vi "Coward.vi"(8 "error in (no error)":errorcluster, 10 "Map":i32[](array[numeric]), 11 "Mother In":refnum<class "Mother.lvclass">) -> (0 "error out":errorcluster, 1 "Direction":T1, 2 "Action":T2, 3 "Mother Out":refnum<class "Mother.lvclass">, 4 "Replicated":refnum<class "Runner.lvclass">)   [LabVIEW 2014, in "Mother.lvclass"]
uses:
  Mother.lvclass
  Action Enum.ctl
  Direction Enum.ctl
  Runner.lvclass
  Coward/Coward.lvclass
  Attack Options.ctl
  Mother.lvclass/Mother.ctl
  SquareBattle.lvclass
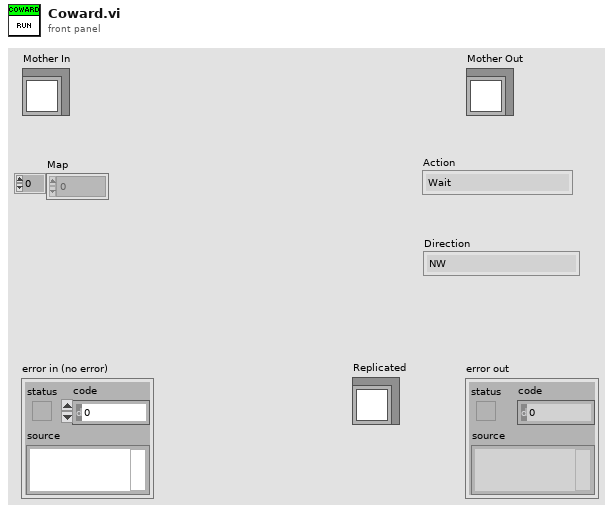
[diagram p1: front panel]
types:
  T1 = typedef "SquareBattle.lvclass/Direction Enum.ctl" = enum16{"NW", "N", "NE", "E", "SE", "S", "SW", "W"}
  T2 = typedef "SquareBattle.lvclass/Action Enum.ctl" = enum16{"Wait", "Move", "Attack", "Replicate"}
  T3 = typedef "Mother.lvclass/Attack Options.ctl" = enum16{"Attack", "Run", "Distract"}
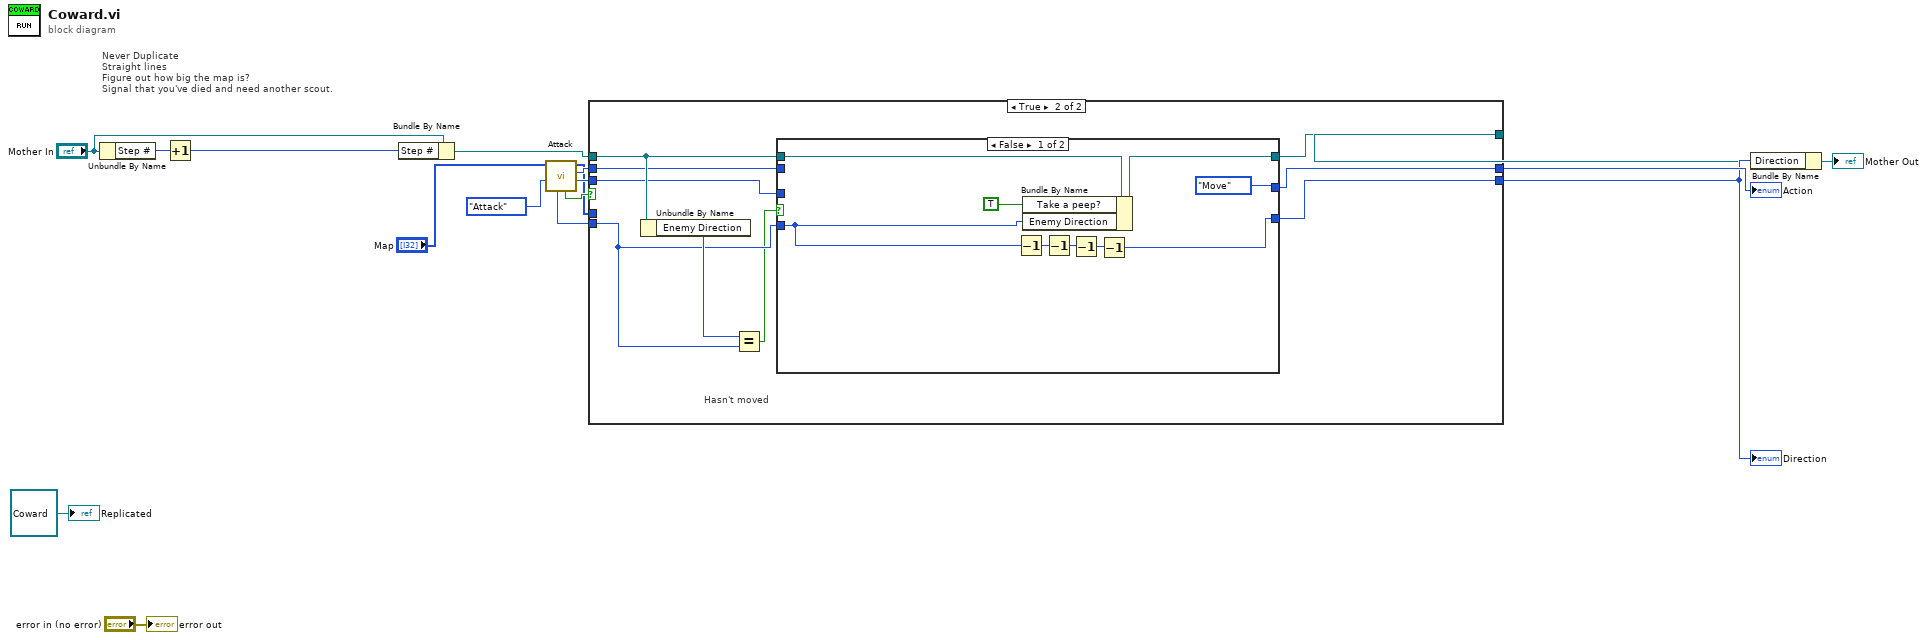
[diagram p0: block diagram]
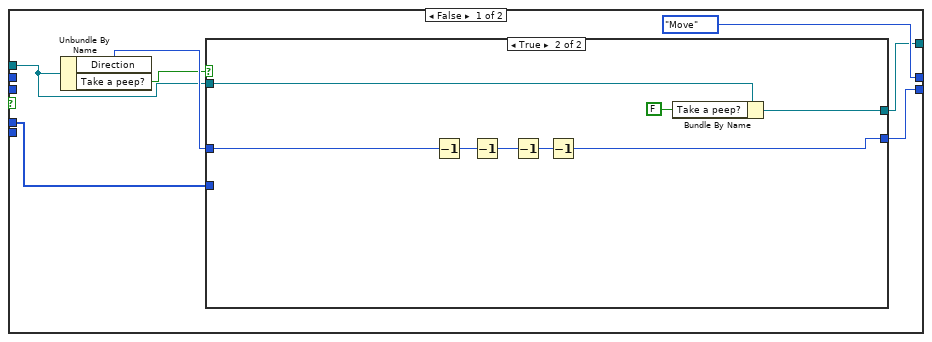
[diagram p2: hidden frame]
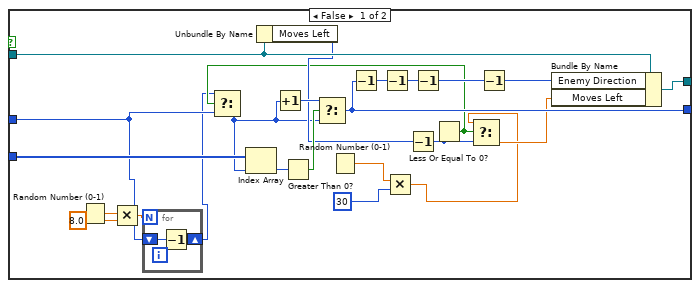
[diagram p3: hidden frame]
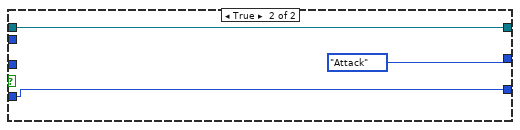
[diagram p4: hidden frame]
diagram:
  # "Never Duplicate\nStraight lines\nFigure out how big the map is?\nSignal that you've died and need another scout."
  n1 = Unbundle By Name("Mother In") -> ("Step #"=w6:i32)
  n2 = Increment(x=w6) -> (x+1=w14:i32)
  n3 = Bundle By Name(cluster="Mother In", "Step #"=w14) -> (w3:refnum<class "Mother.lvclass">)
  n4 = call "Attack.vi"("Attack?"=Attack_Options."Attack", "Maze (0: Empty, -1: Enemy. >0: Teammate"="Map") -> ("Direction"=w8:T1, "Action"=w10:T2, "Maze (0: Empty, -1: Enemy. >0: Teammate 2"=w2:i32[], "Enemy Found?"=w11:bool, "Enemy Direction"=w4:T1)  [unwired: 4 in, 1 out]
  n5 = case shown="True" w11 {
    tunnel: w10 -> [_ w64]
    tunnel: [Action_Enum."Move" ("Action") w63] -> w9
    tunnel: w8 -> [_ w65]
    tunnel: [w23 w62] -> w7
    tunnel: w2 -> [w22 _]
    tunnel: w3 -> [w19 w66]
    tunnel: [w18 w67] -> w5
    tunnel: w4 -> [_ w60]
    frame False {
      n6 = Unbundle By Name(w19) -> ("Direction"=w21:T1, "Take a peep?"=w20:bool)
      n7 = case shown="True" w20 {
        tunnel: [w43 w54] -> w23
        tunnel: w22 -> [w48 _]
        tunnel: w21 -> [w29 w58]
        tunnel: w19 -> [w38 w53]
        tunnel: [w44 w52] -> w18
        frame False {
          n8 = Random Number (0-1)() -> (number: 0 to 1=w34:dbl)
          n9 = Multiply(x=w34, y=8.0) -> (x*y=w30:dbl)
          n10 = for {
            N: w30 -> [_]
            shift-right: [w49] -> w28
            shift-left: w29 -> [w50]
            n11 = Decrement(x=w50) -> (x-1=w49:T1)
          }
          n12 = Unbundle By Name(w38) -> ("Moves Left"=w37:i32)
          n13 = Random Number (0-1)() -> (number: 0 to 1=w27:dbl)
          n14 = Multiply(x=w27, y=30 ("t")) -> (x*y=w25:dbl)
          n15 = Decrement(x=w37) -> (x-1=w35:i32)
          n16 = Less Or Equal To 0?(x=w35) -> (x <= 0?=w31:bool)
          n17 = Select(t=w28, s=w31, f=w29) -> (s? t:f=w32:T1)
          n18 = Index Array(array=w48, index=w32) -> (element=w47:i32)
          n19 = Increment(x=w32) -> (x+1=w45:T1)
          n20 = Greater Than 0?(x=w47) -> (x > 0?=w46:bool)
          n21 = Select(t=w45, s=w46, f=w32) -> (s? t:f=w43:T1)
          n22 = Decrement(x=w43) -> (x-1=w42:T1)
          n23 = Decrement(x=w42) -> (x-1=w41:T1)
          n24 = Decrement(x=w41) -> (x-1=w40:T1)
          n25 = Select(t=w25, s=w31, f=w35) -> (s? t:f=w36:dbl)
          n26 = Decrement(x=w40) -> (x-1=w39:T1)
          n27 = Bundle By Name(cluster=w38, "Enemy Direction"=w39, "Moves Left"=w36) -> (w44:refnum<class "Mother.lvclass">)
        }
        frame True {
          n28 = Decrement(x=w58) -> (x-1=w57:T1)
          n29 = Decrement(x=w57) -> (x-1=w56:T1)
          n30 = Decrement(x=w56) -> (x-1=w55:T1)
          n31 = Decrement(x=w55) -> (x-1=w54:T1)
          n32 = Bundle By Name(cluster=w53, "Take a peep?"=FALSE) -> (w52:refnum<class "Mother.lvclass">)
        }
      }
    }
    frame True {
      # "Hasn't moved"
      n33 = Unbundle By Name(w66) -> ("Enemy Direction"=w61:T1)
      n34 = Equal?(x=w61, y=w60) -> (x = y?=w59:bool)
      n35 = case shown="False" w59 {
        tunnel: [w76 w79] -> w67
        tunnel: w66 -> [w74 w79]
        tunnel: w65 -> [_ _]
        tunnel: w64 -> [_ _]
        tunnel: [Action_Enum."Move" ("Action") Action_Enum."Attack" ("Action")] -> w63
        tunnel: [w69 w77] -> w62
        tunnel: w60 -> [w70 w77]
        frame False {
          n36 = Decrement(x=w70) -> (x-1=w73:T1)
          n37 = Bundle By Name(cluster=w74, "Take a peep?"=TRUE, "Enemy Direction"=w70) -> (w76:refnum<class "Mother.lvclass">)
          n38 = Decrement(x=w73) -> (x-1=w71:T1)
          n39 = Decrement(x=w71) -> (x-1=w72:T1)
          n40 = Decrement(x=w72) -> (x-1=w69:T1)
        }
        frame True {
        }
      }
    }
  }
  "Action" <- w9
  "Direction" <- w7
  n41 = Bundle By Name(cluster=w5, "Direction"=w7) -> (→"Mother Out":refnum<class "Mother.lvclass">)
  "error out" <- "error in (no error)"
  "Replicated" <- refnum<class "Coward.lvclass"> refnum ("Replicated")
